vi "Runtime Test.vi"() -> ()   [LabVIEW 2014, in "FPGA Module tests.lvlib"]
doc: "This VI shows an example for how to test the Runtime functionality of the module. This will need to be modified according to module functionality."
uses:
  FPGA Module tests.lvlib
  module/execution/FPGA Module runtime.lvclass
  <vilib>/NI/Tag Bus/dictionary/data dictionary.lvclass
  <vilib>/NI/Tag Bus/table/data table.lvlib
  module/configuration/FPGA Module configuration.lvclass
  <vilib>/userdefined/High Color/nirio_resource_hc.ctl
  <vilib>/NI/Tag Bus Module Framework/FPGA manager/methods.ctl
  <vilib>/NI/Tag Bus Module Framework/FPGA manager/FPGA manager.lvlib
  <vilib>/rvi/interface/nirviOpenFPGA/nirviOpenFPGA.xnode
  <vilib>/NI/LVFPGA Adv Session Resources/LVFPGAAdvSessionResources.lvlib
  source/FPGA Bitfiles/FPGAModule_FPGATarget_FGPAMaintest_k3awjUENabM.lvbitx
  source/testing/FGPA_Main_test.vi
  <vilib>/FPGAPlugInAG/cRIO-9068/niLvFpga_Open_cRIO-9068.vi
  <vilib>/rvi/interface/common/dynamic/niFpgaDynamicAddResources.vi
  <vilib>/NI/Tag Bus/dictionary/lookup polymorphs/locate Single.vi
  <vilib>/NI/Tag Bus/table/data polymorphs/write one/write Single.vi
  <vilib>/NI/Tag Bus/table/data polymorphs/read one/read Single.vi
  <vilib>/NI/Tag Bus/table/data polymorphs/write one/write Double.vi
  <vilib>/NI/Tag Bus/dictionary/lookup polymorphs/locate double.vi
  <vilib>/NI/Tag Bus/table/data polymorphs/write one/write I32.vi
  <vilib>/NI/Tag Bus/table/data polymorphs/write one/write Boolean.vi
  <vilib>/NI/Tag Bus/dictionary/lookup polymorphs/locate I32.vi
  <vilib>/NI/Tag Bus/dictionary/lookup polymorphs/locate Boolean.vi
  <vilib>/NI/Tag Bus/table/data polymorphs/read one/read I32.vi
  <vilib>/NI/Tag Bus/table/data polymorphs/read one/read Double.vi
  <vilib>/NI/Tag Bus/table/data polymorphs/read one/read Boolean.vi
  <vilib>/NI/LVFPGA Adv Session Resources/ResourceInfo.ctl
panel:
  out "Boolean Match":bool
  out "Double Match":bool
  out "I32 Match":bool
  out "Resource info out":T1[](array[typedef])
  out "final error":errorcluster
  out "output error":errorcluster
  out "input error":errorcluster
  out "Single Match":bool
  out "init error":errorcluster
  out "correct execution settings":bool
  out "invalid configuration":errorcluster
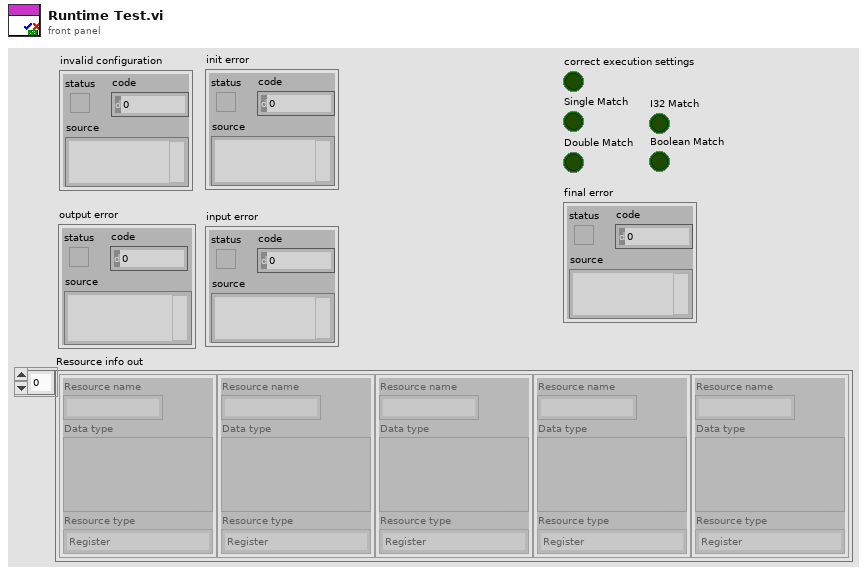
[diagram p1: front panel]
types:
  T1 = typedef "LVFPGAAdvSessionResources.lvlib/ResourceInfo.ctl" = cluster{"Resource name":string, "Data type":variant, "Resource type":enum16{"Register", "Host To Target FIFO", "Target To Host FIFO"}}
  T2 = typedef "FPGA manager.lvlib/methods.ctl" = enum16{"initialize bitfile", "cache bitfile", "locate bitfile", "close bitfile", "clear manager"}
  T3 = typedef "nirio_resource_hc.ctl" = tag
  T4 = typedef "TBM channel.lvclass/data tables.ctl" = cluster{"input data":T5, "processing parameter":T5, "processing result":T5, "output data":T5}
  T5 = typedef "tag bus.lvlib/dictionary table pair.ctl" = cluster{"data dictionary":refnum<class "data dictionary.lvclass">, "data table":T6}
  T6 = typedef "tag bus.lvlib/data table.lvlib/data table.ctl" = cluster{"Double":dbl[], "Single":sgl[], "I64":i64[], "I32":i32[], "I16":i16[], "I8":i8[], "U64":u64[], "U32":u32[], "U16":u16[], "U8":u8[], "Boolean":bool[], "String":string[], "Array of Double":cluster{"DBL Array":dbl[]}[], "Array of Single":cluster{"SGL Array":sgl[]}[], "Array of I64":cluster{"I64 Array":i64[]}[], "Array of I32":cluster{"I32 Array":i32[]}[], "Array of I16":cluster{"I16 Array":i16[]}[], "Array of I8":cluster{"I8 Array":i8[]}[], "Array of U64":cluster{"U64 Array":u64[]}[], "Array of U32":cluster{"U32 Array":u32[]}[], "Array of U16":cluster{"U16 Array":u16[]}[], "Array of U8":cluster{"U8 Array":u8[]}[], "Array of Boolean":cluster{"Boolean Array":bool[]}[], "Array of String":cluster{"String Array":string[]}[]}
  T7 = typedef "TBM module execution interface.lvclass/execution settings.ctl" = cluster{"reads inputs":bool, "processes data":bool, "writes outputs":bool}
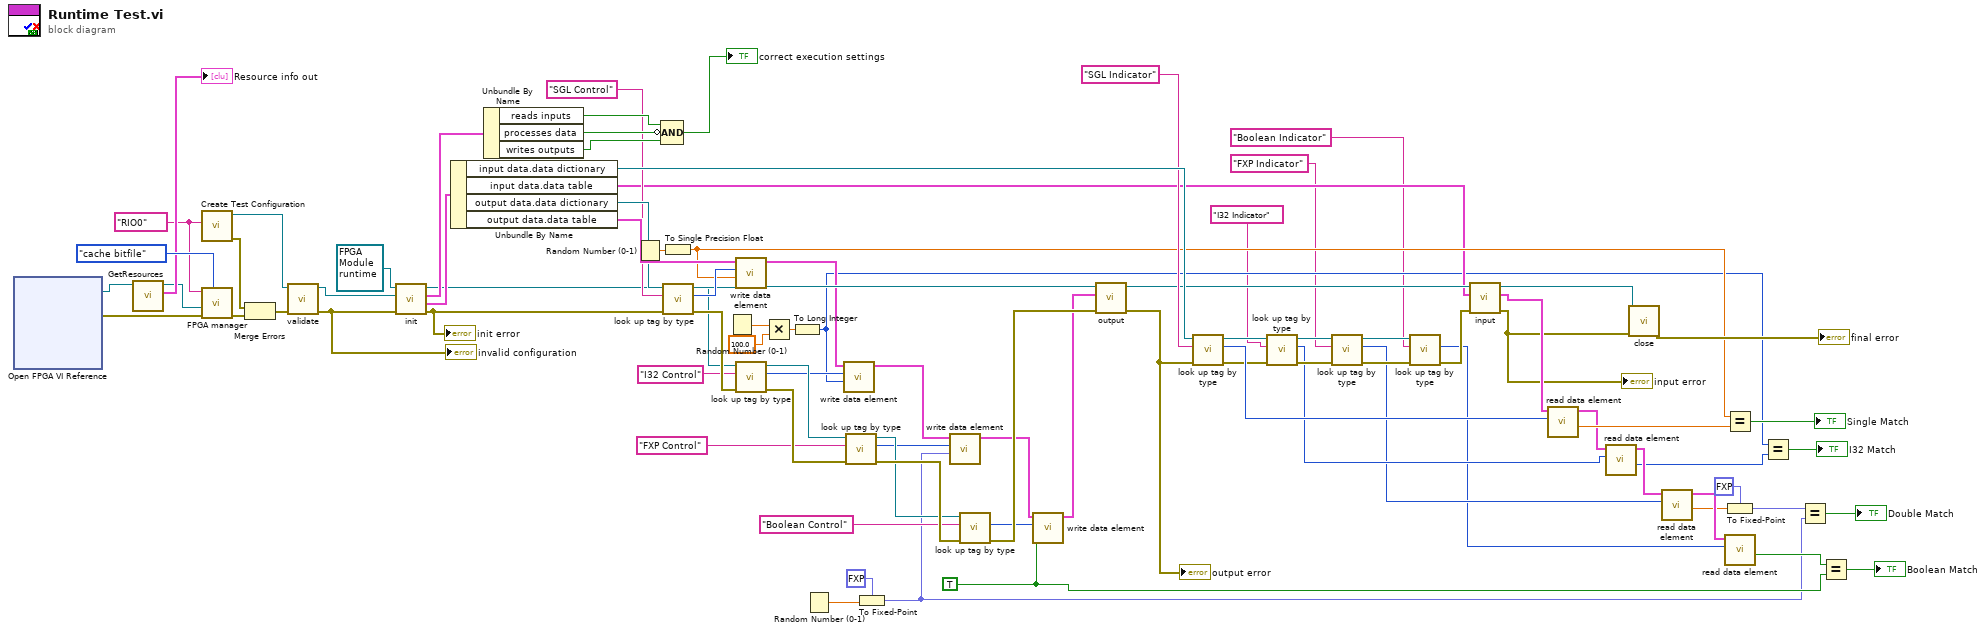
[diagram p0: block diagram]
diagram:
  w10 = TRUE ("value")
  w64 = T3 "RIO0" ("RIO resource")
  n1 = xnode "Open FPGA VI Reference"() -> ("FPGA VI Reference Out"=w67:refnum<k20>, "error out"=w70:errorcluster)  [unwired: 2 in]
  n2 = call <vilib>:"GetResources.vi"("FPGA VI Reference in"=w67) -> ("Resource info out"=→"Resource info out":T1[], "FPGA VI Reference out"=w65:refnum<k20>)  [unwired: 8 in, 1 out]
  n3 = call "Create Test Configuration.vi"("RIO Device"=w64) -> ("error out"=w72:errorcluster, "Module Configuration"=w73:refnum<class "FPGA Module configuration.lvclass">)  [unwired: 5 in, 4 out]
  n4 = call <vilib>:"FPGA manager.vi"("action"=methods."cache bitfile", "error in"=w70, "bitfile to cache"=w65, "RIO resource"=w64) -> ("error out"=w68:errorcluster)  [unwired: 5 in, 2 out]
  n5 = Merge Errors(w72, w68) -> (w71:errorcluster)
  n6 = call-dynamic "validate.vi"("error in"=w71, "FPGA Module configuration in"=w73) -> ("error out"=w87:errorcluster, "FPGA Module configuration out"=w88:refnum<class "FPGA Module configuration.lvclass">)  [unwired: 8 in]
  "invalid configuration" <- w87
  n7 = call-dynamic "init.vi"("error in"=w87, "TBM module configuration in"=w88, "FPGA Module runtime in"=refnum<class "FPGA Module runtime.lvclass"> refnum ("tag bus configurable plugin module")) -> ("error out"=w56:errorcluster, "data allocations"=w80:T4, "execution settings"=w85:T7, "FPGA Module runtime out"=w60:refnum<class "FPGA Module runtime.lvclass">)  [unwired: 5 in]
  "init error" <- w56
  n8 = Unbundle By Name(w80) -> ("input data.data dictionary"=w79:refnum<class "data dictionary.lvclass">, "input data.data table"=w27:T6, "output data.data dictionary"=w63:refnum<class "data dictionary.lvclass">, "output data.data table"=w75:T6)
  n9 = Unbundle By Name(w85) -> ("reads inputs"=w82:bool, "processes data"=w84:bool, "writes outputs"=w83:bool)
  n10 = Random Number (0-1)() -> (number: 0 to 1=w52:dbl)
  n11 = Compound Arithmetic op=AND(w82, invert w84, w83) -> (→"correct execution settings":bool)
  n12 = To Single Precision Float(number=w52) -> (single precision float=w51:sgl)
  n13 = call-poly <vilib>:"look up tag by type.vi"("error in"=w56, "name"="SGL Control", "data dictionary in"=w63) -> ("error out"=w49:errorcluster, "index"=w61:i32, "data dictionary out"=w45:refnum<class "data dictionary.lvclass">)  [unwired: 6 in]
  n14 = Random Number (0-1)() -> (number: 0 to 1=w32:dbl)
  n15 = call-poly <vilib>:"write data element.vi"("value"=w51, "index"=w61, "data table in"=w75) -> ("data table out"=w39:T6)  [unwired: 8 in]
  n16 = call-poly <vilib>:"look up tag by type.vi"("error in"=w49, "name"="I32 Control", "data dictionary in"=w45) -> ("error out"=w50:errorcluster, "index"=w40:i32, "data dictionary out"=w44:refnum<class "data dictionary.lvclass">)  [unwired: 6 in]
  n17 = Multiply(x=w32, y=100.0) -> (x*y=w31:dbl)
  n18 = To Long Integer(number=w31) -> (32bit integer=w13:i32)
  n19 = Random Number (0-1)() -> (number: 0 to 1=w5:dbl)
  n20 = call-poly <vilib>:"write data element.vi"("value"=w13, "index"=w40, "data table in"=w39) -> ("data table out"=w38:T6)  [unwired: 8 in]
  n21 = call-poly <vilib>:"look up tag by type.vi"("error in"=w50, "name"="FXP Control", "data dictionary in"=w44) -> ("error out"=w48:errorcluster, "index"=w35:i32, "data dictionary out"=w43:refnum<class "data dictionary.lvclass">)  [unwired: 6 in]
  n22 = To Fixed-Point(fixed-point type=fxp<+/-,20,5> 0.0 ("FXP Control"), number=w5) -> (fixed-point=w4:fxp<+/-,20,5>)
  n23 = call-poly <vilib>:"write data element.vi"("value"=w4, "index"=w35, "data table in"=w38) -> ("data table out"=w37:T6)  [unwired: 8 in]
  n24 = call-poly <vilib>:"look up tag by type.vi"("error in"=w48, "name"="Boolean Control", "data dictionary in"=w43) -> ("error out"=w47:errorcluster, "index"=w34:i32)  [unwired: 6 in, 1 out]
  n25 = call-poly <vilib>:"write data element.vi"("value"=w10, "index"=w34, "data table in"=w37) -> ("data table out"=w36:T6)  [unwired: 8 in]
  n26 = call-dynamic "output.vi"("error in"=w47, "data table in"=w36, "FPGA Module runtime in"=w60) -> ("error out"=w55:errorcluster, "FPGA Module runtime out"=w58:refnum<class "FPGA Module runtime.lvclass">)  [unwired: 6 in, 1 out]
  "output error" <- w55
  n27 = call-poly <vilib>:"look up tag by type.vi"("error in"=w55, "name"="SGL Indicator", "data dictionary in"=w79) -> ("error out"=w26:errorcluster, "index"=w77:i32, "data dictionary out"=w28:refnum<class "data dictionary.lvclass">)  [unwired: 6 in]
  n28 = call-poly <vilib>:"look up tag by type.vi"("error in"=w26, "name"="I32 Indicator", "data dictionary in"=w28) -> ("error out"=w25:errorcluster, "index"=w19:i32, "data dictionary out"=w29:refnum<class "data dictionary.lvclass">)  [unwired: 6 in]
  n29 = call-poly <vilib>:"look up tag by type.vi"("error in"=w25, "name"="FXP Indicator", "data dictionary in"=w29) -> ("error out"=w24:errorcluster, "index"=w18:i32, "data dictionary out"=w30:refnum<class "data dictionary.lvclass">)  [unwired: 6 in]
  n30 = call-poly <vilib>:"look up tag by type.vi"("error in"=w24, "name"="Boolean Indicator", "data dictionary in"=w30) -> ("error out"=w23:errorcluster, "index"=w17:i32)  [unwired: 6 in, 1 out]
  n31 = call-dynamic "input.vi"("error in"=w23, "data table in"=w27, "FPGA Module runtime in"=w58) -> ("error out"=w53:errorcluster, "data table out"=w78:T6, "FPGA Module runtime out"=w57:refnum<class "FPGA Module runtime.lvclass">)  [unwired: 6 in]
  "input error" <- w53
  n32 = call-poly <vilib>:"read data element.vi"("index"=w77, "data table in"=w78) -> ("value"=w54:sgl, "data table out"=w22:T6)  [unwired: 8 in]
  n33 = call-poly <vilib>:"read data element.vi"("index"=w19, "data table in"=w22) -> ("value"=w12:i32, "data table out"=w21:T6)  [unwired: 8 in]
  n34 = call-dynamic "close.vi"("error in"=w53, "FPGA Module runtime in"=w57) -> ("error out"=→"final error":errorcluster)  [unwired: 9 in]
  n35 = call-poly <vilib>:"read data element.vi"("index"=w18, "data table in"=w21) -> ("value"=w2:dbl, "data table out"=w20:T6)  [unwired: 8 in]
  n36 = Equal?(x=w51, y=w54) -> (x = y?=→"Single Match":bool)
  n37 = To Fixed-Point(fixed-point type=fxp<+/-,20,5> 0.0 ("FXP Control"), number=w2) -> (fixed-point=w1:fxp<+/-,20,5>)
  n38 = call-poly <vilib>:"read data element.vi"("index"=w17, "data table in"=w20) -> ("value"=w11:bool)  [unwired: 8 in, 1 out]
  n39 = Equal?(x=w13, y=w12) -> (x = y?=→"I32 Match":bool)
  n40 = Equal?(x=w1, y=w4) -> (x = y?=→"Double Match":bool)
  n41 = Equal?(x=w11, y=w10) -> (x = y?=→"Boolean Match":bool)
